vi "ADI_IMU_ADIS16470_ReadSensorData.vi"(8 "error in (no error)":errorcluster, 11 "SPIDevRef in":T1) -> (0 "error out":errorcluster, 2 "Data Array":dbl[](array[numeric]), 3 "SPIDevRef out":T1)   [LabVIEW 2017, in "ADIS16470_IMU.lvlib"]
uses:
  ADIS16470_IMU.lvlib
  <vilib>/Rock Robotics/WPI/SPI/WPI_SPIDevRef.ctl
  <vilib>/Rock Robotics/SystemInterfaces/spilib/spi_bus.ctl
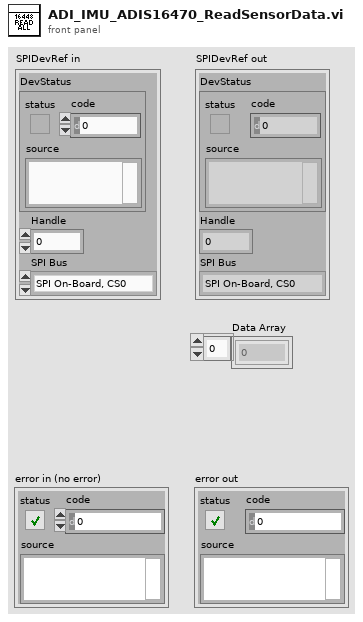
[diagram p1: front panel]
types:
  T1 = typedef "WPI_SPIDevRef.ctl" = cluster{"DevStatus":errorcluster, "Handle":i32, "SPI Bus":T2}
  T2 = typedef "spi_bus.ctl" = enum16{"SPI On-Board, CS0", "SPI On-Board, CS1", "SPI On-Board, CS2", "SPI On-Board, CS3", "SPI MXP", "Invalid"}
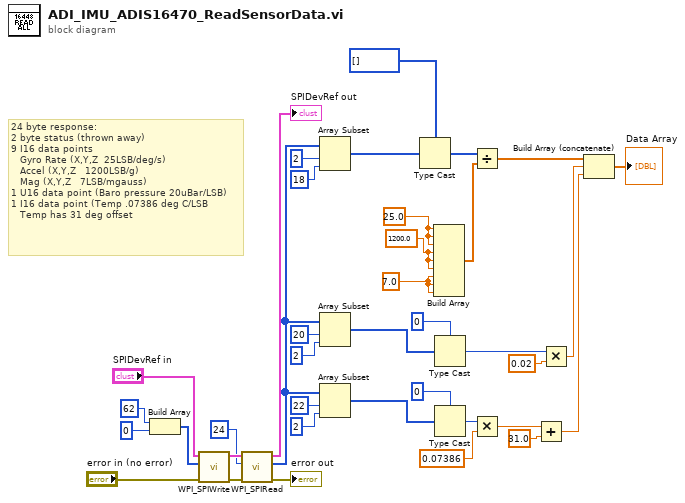
[diagram p0: block diagram]
diagram:
  w34 = 7.0
  w35 = 1200.0
  w36 = 25.0 ("element")
  # "24 byte response:\n2 byte status (thrown away)\n9 I16 data points\n   Gyro Rate (X,Y,Z  25LSB/deg/s)\n   Accel (X,Y,Z   1200LSB/g)\n   Mag (X,Y,Z   7LSB/mgauss)\n1 U16 data point (Baro pressure 20uBar/LSB)\n1 I16 data point (Temp .07386 deg C/LSB\n   Temp has 31 deg offset"
  n1 = Build Array(u8 62 ("hi"), u8 0 ("lo")) -> (w30:u8[])
  n2 = call <vilib>:"WPI_SPIWrite.vi"("error in (no error)"="error in (no error)", "Data To Send"=w30, "SPIDevRef"="SPIDevRef in") -> ("error out"=w29:errorcluster, "SPIDevRef"=w28:T1)  [unwired: 7 out]
  n3 = call <vilib>:"WPI_SPIRead.vi"("error in (no error)"=w29, "Num to Read"=24, "SPIDevRef"=w28) -> ("error out"=→"error out":errorcluster, "Received Data"=w7:u8[], "SPIDevRef"=→"SPIDevRef out":T1)  [unwired: 6 in]
  n4 = Array Subset(array=w7, index=2, length=18) -> (w3:u8[])
  n5 = Array Subset(array=w7, index=20, length=2) -> (w10:u8[])
  n6 = Array Subset(array=w7, index=22, length=2) -> (w8:u8[])
  n7 = Type Cast(type=i16[] [], x=w3) -> (*(type *) &x=w1:i16[])
  n8 = Build Array(w36, w36, w36, w35, w35, w35, w34, w34, w34) -> (w33:dbl[])
  n9 = Type Cast(type=u16 0, x=w10) -> (*(type *) &x=w5:u16)
  n10 = Type Cast(type=i16 0, x=w8) -> (*(type *) &x=w4:i16)
  n11 = Divide(x=w1, y=w33) -> (x/y=w20:dbl[])
  n12 = Multiply(x=w4, y=0.07386 ("element")) -> (x*y=w22:dbl)
  n13 = Add(x=w22, y=31.0) -> (x+y=w19:dbl)
  n14 = Multiply(x=w5, y=0.02) -> (x*y=w17:dbl)
  n15 = Build Array (concatenate)(w20, w17, w19) -> (→"Data Array":dbl[])
